vi "DistanceCalculator.vi"(10 "Number2":i32, 11 "Number1":i32) -> (3 "Distance":i32)   [LabVIEW 2017]
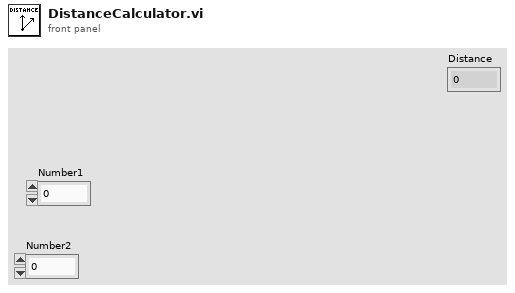
[diagram p1: front panel]
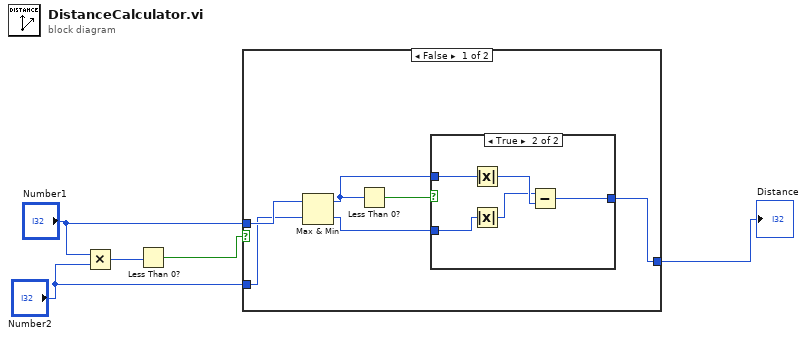
[diagram p0: block diagram]
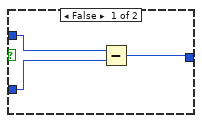
[diagram p2: hidden frame]
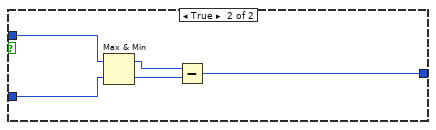
[diagram p3: hidden frame]
diagram:
  n1 = Multiply(x="Number1", y="Number2") -> (x*y=w4:i32)
  n2 = Less Than 0?(x=w4) -> (x < 0?=w5:bool)
  n3 = case shown="False" w5 {
    tunnel: "Number2" -> [w9 w24]
    tunnel: "Number1" -> [w10 w23]
    tunnel: [w8 w20] -> w1
    frame False {
      n4 = Max & Min(x=w10, y=w9) -> (max(x,y)=w7:i32, min(x,y)=w6:i32)
      n5 = Less Than 0?(x=w7) -> (x < 0?=w11:bool)
      n6 = case shown="True" w11 {
        tunnel: w7 -> [w14 w19]
        tunnel: w6 -> [w13 w18]
        tunnel: [w12 w17] -> w8
        frame False {
          n7 = Subtract(x=w14, y=w13) -> (x-y=w12:i32)
        }
        frame True {
          n8 = Absolute Value(x=w19) -> (abs(x)=w16:i32)
          n9 = Absolute Value(x=w18) -> (abs(x)=w15:i32)
          n10 = Subtract(x=w15, y=w16) -> (x-y=w17:i32)
        }
      }
    }
    frame True {
      n11 = Max & Min(x=w23, y=w24) -> (max(x,y)=w22:i32, min(x,y)=w21:i32)
      n12 = Subtract(x=w22, y=w21) -> (x-y=w20:i32)
    }
  }
  "Distance" <- w1
